vi "Log GlobalStop.WriterState.vi"(8 "error in":errorcluster) -> (0 "error out":errorcluster)   [LabVIEW 2021, in "XNET-CAN-Signal-Logger.lvlib"]
uses:
  XNET-CAN-Signal-Logger.lvlib
  Global Variables.vi
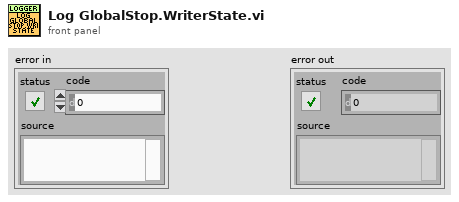
[diagram p1: front panel]
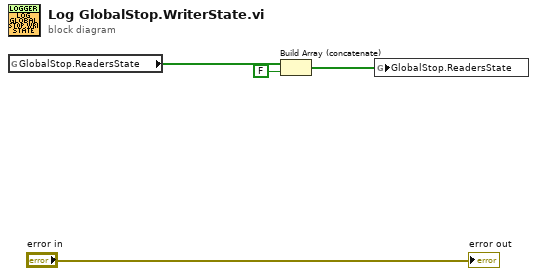
[diagram p0: block diagram]
diagram:
  n1 = global read "Global Variables.vi" "GlobalStop.ReadersState"() -> (w4:bool[])
  n2 = Build Array (concatenate)(w4, FALSE ("Boolean")) -> (w2:bool[])
  n3 = global write "Global Variables.vi" "GlobalStop.ReadersState"(w2) -> ()
  "error out" <- "error in"
